vi "_ButtonGroupEnum to Num.vi"(5 "Enum":variant, 8 "error in":errorcluster, 9 "Prefix":string, 11 "CtlRef":refnum<vi>) -> (0 "error out":errorcluster, 2 "num":i32, 3 "CtlRef (dup)":refnum<vi>)   [LabVIEW 2017, in "ButtonGroupEnum.lvlib"]
uses:
  ButtonGroupEnum.lvlib
  _openG/_reuse_openG.lvlib
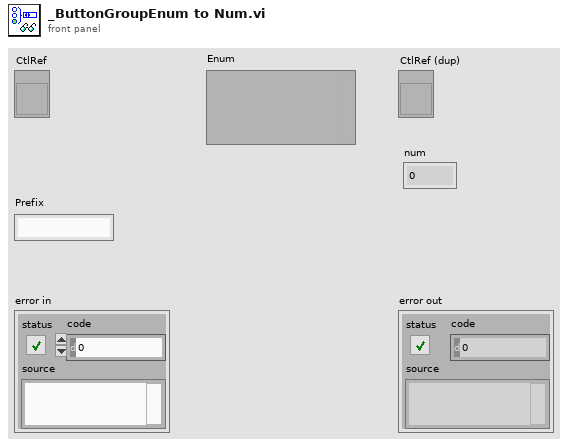
[diagram p1: front panel]
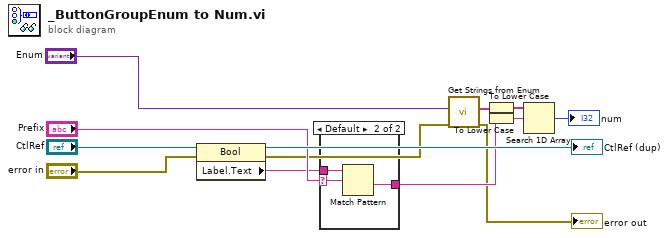
[diagram p0: block diagram]
diagram:
  n1 = property class="Bool"(reference="CtlRef", error in="error in") -> (reference out=→"CtlRef (dup)":refnum<vi>, error out=w6:errorcluster, "Label.Text"=w8:string)
  n2 = case shown="Default" "Prefix" {
    selector: "Prefix" -> [_ w16]
    tunnel: w8 -> [w14 w17]
    tunnel: [w14 w15] -> w3
    frame "" {
    }
    frame Default {
      n3 = Match Pattern(string=w17, regular expression=w16) -> (after substring=w15:string)  [unwired: 1 in, 3 out]
    }
  }
  n4 = call "Get Strings from Enum.vi"("error in (no error)"=w6, "Enum"="Enum") -> ("error out"=→"error out":errorcluster, "Enum Strings"=w5:string[])  [unwired: 6 in, 2 out]
  n5 = To Lower Case(string=w5) -> (all lower case string=w4:string[])
  n6 = To Lower Case(string=w3) -> (all lower case string=w7:string)
  n7 = Search 1D Array(1D array=w4, element=w7) -> (index of element=→"num":i32)  [unwired: 1 in]
